vi "WSVCAP SHL FPGA LL Procedure SPI - Send Receive.vi"(0 "Procedure Step":T1, 1 "Wait Ticks Remaining":u32, 2 "CMD Length [1-40]":u8, 5 "SPI Wait Ticks":u32, 7 "Write Bit Index [0-39]":u8, 9 "SPI Cycle Mode":bool, 11 "error in (no error)":errorcluster, 12 "SPI Cycle CMD":u64, 13 "Socket Mask":u32) -> (3 "Wait Ticks Remaining Out":u32, 4 "Procedure Step Out":T1, 8 "Write Bit Index [0-39] Out":u8, 10 "Finished":bool, 15 "error out":errorcluster)   [LabVIEW 2012]
uses:
  Type Defs/WSVCAP SHL Procedure Step Enum.ctl
  Type Defs/WSVCAP SHL SPI Write Line Enum.ctl
  Type Defs/WSVCAP SHL FIFO Operation Enum.ctl
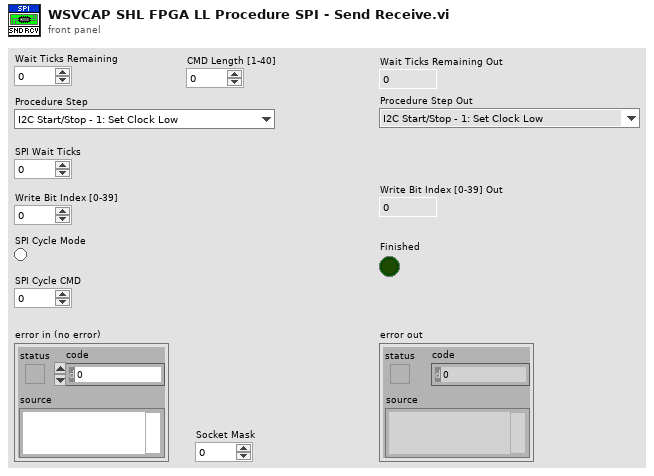
[diagram p1: front panel]
types:
  T1 = typedef "WSVCAP SHL Procedure Step Enum.ctl" = enum16{"I2C Start/Stop - 1: Set Clock Low", "I2C Start/Stop - 2: Wait", "I2C Start/Stop - 3: Set Data I", "I2C Start/Stop - 4: Wait", "I2C Start/Stop - 5: Set Clock High", "I2C Start/Stop - 6: Wait", "I2C Start/Stop - 7: Set Data II", "I2C Start/Stop - 8: Wait", "I2C Start/Stop - 9: Set Clock Low", "I2C Start/Stop - 10: Wait", "I2C Read ACK - 1: Set Clock High", "I2C Read ACK - 2: Wait", "I2C Read ACK - 3: Read ACK Bit", "I2C Read ACK - 4: Wait", "I2C Read ACK - 5: Set Clock Low", "I2C Read ACK - 6: Wait", "I2C Write ACK - 1: Write ACK Bit", "I2C Write ACK - 2: Wait", "I2C Write ACK - 3: Set Clock High", "I2C Write ACK - 4: Wait", "I2C Write ACK - 5: Set Clock Low", "I2C Write ACK - 6: Wait", "I2C Write ACK - 7: Set Data Low", "I2C Send Add - 1: Reset Bits Remaining", "I2C Send Add - 2: Set Data Bit", "I2C Send Add - 3: Wait", "I2C Send Add - 4: Set Clock High", "I2C Send Add - 5: Wait", "I2C Send Add - 6: Set Clock Low", "I2C Send Add - 7: Wait", "I2C Send Add - 8: Check Bits Remaining", "I2C Send Data - 1: Reset Bits Remaining", "I2C Send Data - 2: Load Write Bit from FIFO", "I2C Send Data - 3: Set Data Bit", "I2C Send Data - 4: Wait", "I2C Send Data - 5: Set Clock High", "I2C Send Data - 6: Wait", "I2C Send Data - 7: Set Clock Low", "I2C Send Data - 8: Wait", "I2C Send Data - 9: Check Bits Remaining", "I2C Receive Data - 1: Reset Bits Remaining", "I2C Receive Data - 2: Wait", "I2C Receive Data - 3: Set Clock High", "I2C Receive Data - 4: Wait", "I2C Receive Data - 5: Read Data Bit", "I2C Receive Data - 6: Wait", "I2C Receive Data - 7: Set Clock Low", "I2C Receive Data - 8: Wait", "I2C Receive Data - 9: Check Bits Remaining", "SPI Clear Lines - 1:Clear", "SPI Send/Receive - 1: Load SDA - Clock Low", "SPI Send/Receive - 2: Wait", "SPI Send/Receive - 3: Load DATO - Clock High", "SPI Send/Receive - 4: Wait", "SPI Wait CMD Delay - 1:Wait", "RFFE Send SSC - 1:Set Low", "RFFE Send SSC - 2:Wait", "RFFE Send SSC - 3:Set SDA High", "RFFE Send SSC - 4:Wait", "RFFE Send SSC - 5:Set SDA Low", "RFFE Send SSC - 6:Wait", "RFFE Send Data - 1:Set SCL High", "RFFE Send Data - 2:Wait", "RFFE Send Data - 3:Set SCL Low", "RFFE Send Data - 4:Wait", "RFFE Send Data - 5:Set SCL High (P)", "RFFE Send Data - 6:Wait", "RFFE Send Data - 7:Set SCL Low (P)", "RFFE Send Data - 8:Wait", "RFFE Send Data - 9:Set SCL High (BP)", "RFFE Send Data - 10:Wait", "RFFE Send Data - 11:Set SCL Low (BP)", "RFFE Send Data - 12:Wait", "RFFE Receive Data - 1:Set SCL High", "RFFE Receive Data - 2:Wait", "RFFE Receive Data - 3:Set SCL Low", "RFFE Receive Data - 4:Wait", "RFFE Receive Data - 5:Set SCL High (BP)", "RFFE Receive Data - 6:Wait", "RFFE Receive Data - 7:Set SCL Low (BP)", "RFFE Receive Data - 8:Wait", "RFFE Wait CMD Delay - 1:Wait", "RFFE Clear Lines - 1:Clear"}
  T2 = typedef "WSVCAP SHL SPI Write Line Enum.ctl" = enum16{"SDAA", "SDEN", "SCLK"}
  T3 = typedef "WSVCAP SHL FIFO Operation Enum.ctl" = enum16{"Create FIFO/Memory", "Get Write FIFO Status", "Get Read FIFO Status", "Put Element in Write", "Put Element in Read", "Get Element from Write", "Get Element from Read"}
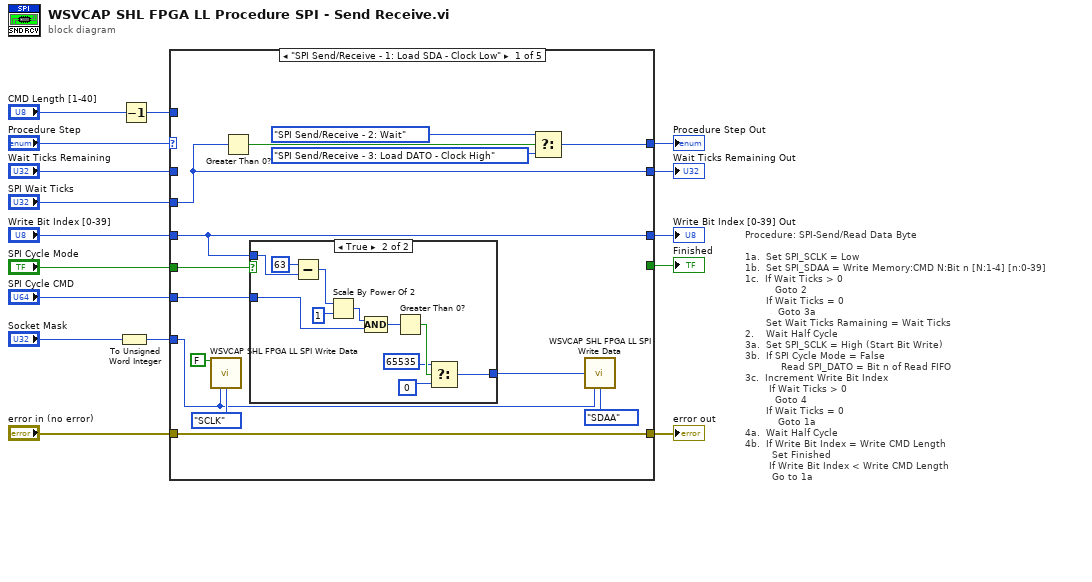
[diagram p0: block diagram]
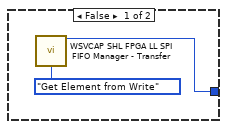
[diagram p2: hidden frame]
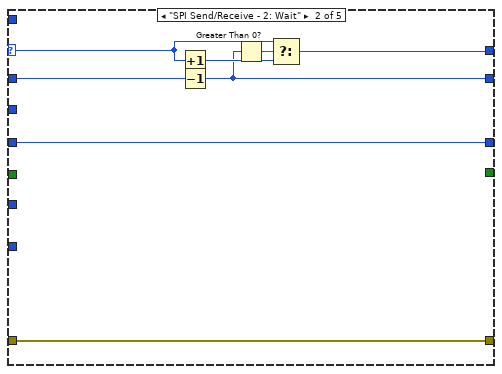
[diagram p3: hidden frame]
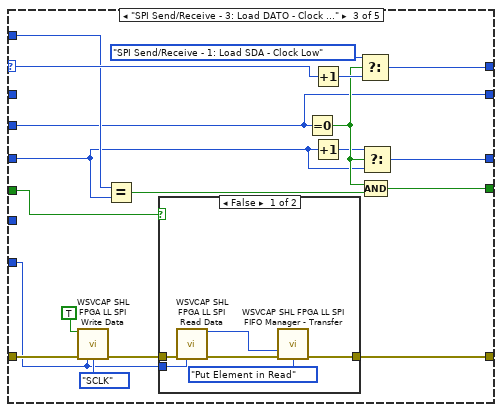
[diagram p4: hidden frame]
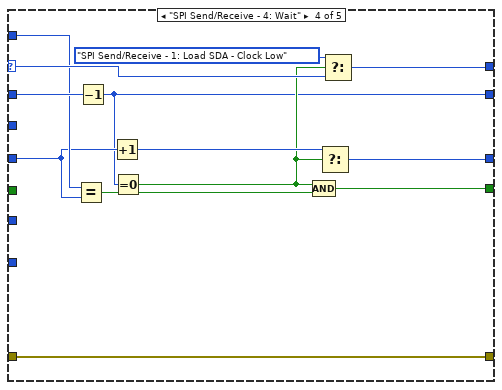
[diagram p6: hidden frame]
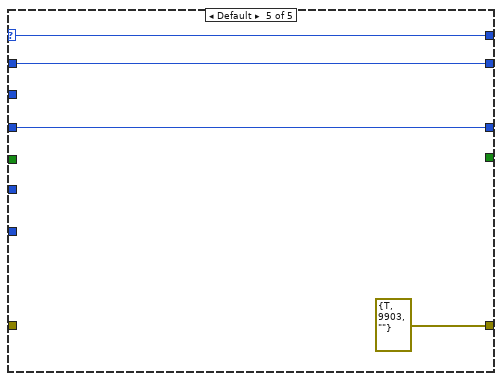
[diagram p7: hidden frame]
diagram:
  # "Procedure: SPI-Send/Read Data Byte\n\n1a.  Set SPI_SCLK = Low\n1b.  Set SPI_SDAA = Write Memory:CMD N:Bit n [N:1-4] [n:0-39]\n1c.  If Wait Ticks > 0\n          Goto 2\n       If Wait Ticks = 0 \n           Goto 3a\n       Set Wait Ticks Ramaining = Wait Ticks\n2.    Wait Half Cycle\n3a.  Set SPI_SCLK = High (Start Bit Write)\n3b.  If SPI Cycle Mode = False\n            Read SPI_DATO = Bit n of Read FIFO            \n3c.  Increment Write Bit Index\n        If Wait Ticks > 0\n          Goto 4\n       If Wait Ticks = 0 \n           Goto 1a \n4a.  Wait Half Cycle\n4b.  If Write Bit Index = Write CMD Length\n         Set Finished\n        If Write Bit Index < Write CMD Length\n         Go to 1a"
  n1 = To Unsigned Word Integer(number="Socket Mask") -> (unsigned 16bit integer=w11:u16)
  n2 = Decrement(x="CMD Length [1-40]") -> (x-1=w10:u8)
  n3 = case shown="\"SPI Send/Receive - 1: Load SDA - Clock Low\"" "Procedure Step" {
    selector: "Procedure Step" -> [_ w49 w70 w89 w93]
    tunnel: [w24 w51 w64 w90 errorcluster {"status"=TRUE, "code"=9903, "source"=""} ("error IO")] -> w15
    tunnel: "error in (no error)" -> [w24 w51 w66 w90 _]
    tunnel: "Wait Ticks Remaining" -> [_ w47 _ w88 w92]
    tunnel: "SPI Wait Ticks" -> [w18 _ w53 _ _]
    tunnel: [_ _ w62 w82 _] -> w14
    tunnel: "Write Bit Index [0-39]" -> [w17 w44 w56 w86 w91]
    tunnel: w11 -> [w26 _ w63 _ _]
    tunnel: "SPI Cycle Mode" -> [w23 _ w61 _ _]
    tunnel: "SPI Cycle CMD" -> [w22 _ _ _ _]
    tunnel: w10 -> [_ _ w60 w87 _]
    tunnel: [w19 w46 w54 w80 w93] -> w3
    tunnel: [w18 w45 w53 w79 w92] -> w2
    tunnel: [w17 w44 w52 w78 w91] -> w1
    frame "SPI Send/Receive - 1: Load SDA - Clock Low" {
      n4 = call "WSVCAP SHL FPGA LL SPI Write Data.vi"("Bit In"=FALSE, "Socket Mask"=w26, "Line"=WSVCAP_SHL_SPI_Write_Line_Enum."SCLK") -> ()  [unwired: 12 in, 1 out]
      n5 = Greater Than 0?(x=w18) -> (x > 0?=w27:bool)
      n6 = case shown="True" w23 {
        tunnel: [w31 w37] -> w25
        tunnel: w22 -> [_ w36]
        tunnel: w17 -> [_ w34]
        frame False {
          n7 = call "WSVCAP SHL FPGA LL SPI FIFO Manager - Transfer.vi"("Operation"=WSVCAP_SHL_FIFO_Operation_Enum."Get Element from Write") -> ("Data Out"=w31:u16)  [unwired: 12 in, 2 out]
        }
        frame True {
          n8 = Subtract(x=u8 63 ("y"), y=w34) -> (x-y=w33:u8)
          n9 = Scale By Power Of 2(n=w33, x=u64 1 ("Data Out")) -> (x*2^n=w42:u64)
          n10 = Compound Arithmetic op=AND(w42, w36) -> (w41:u64)
          n11 = Greater Than 0?(x=w41) -> (x > 0?=w40:bool)
          n12 = Select(t=u16 65535 ("Data Out"), s=w40, f=u16 0 ("Data Out")) -> (s? t:f=w37:u16)
        }
      }
      n13 = Select(t=WSVCAP_SHL_Procedure_Step_Enum."SPI Send/Receive - 2: Wait" ("Procedure Step"), s=w27, f=WSVCAP_SHL_Procedure_Step_Enum."SPI Send/Receive - 3: Load DATO - Clock High" ("Procedure Step")) -> (s? t:f=w19:T1)
      n14 = call "WSVCAP SHL FPGA LL SPI Write Data.vi"("Data Word In"=w25, "Socket Mask"=w26, "Line"=WSVCAP_SHL_SPI_Write_Line_Enum."SDAA") -> ()  [unwired: 12 in, 1 out]
    }
    frame "SPI Send/Receive - 2: Wait" {
      n15 = Increment(x=w49) -> (x+1=w48:T1)
      n16 = Decrement(x=w47) -> (x-1=w45:u32)
      n17 = Greater Than 0?(x=w45) -> (x > 0?=w50:bool)
      n18 = Select(t=w49, s=w50, f=w48) -> (s? t:f=w46:T1)
    }
    frame "SPI Send/Receive - 3: Load DATO - Clock High" {
      n19 = call "WSVCAP SHL FPGA LL SPI Write Data.vi"("Bit In"=TRUE, "error in (no error)"=w66, "Socket Mask"=w63, "Line"=WSVCAP_SHL_SPI_Write_Line_Enum."SCLK") -> ("error out"=w65:errorcluster)  [unwired: 11 in]
      n20 = Equal?(x=w60, y=w56) -> (x = y?=w59:bool)
      n21 = case shown="False" w61 {
        tunnel: w65 -> [w76 w77]
        tunnel: [w73 w77] -> w64
        tunnel: w63 -> [w72 _]
        frame False {
          n22 = call "WSVCAP SHL FPGA LL SPI Read Data.vi"("error in (no error)"=w76, "Socket Mask"=w72) -> ("Word Out (1-Bit for Each Channel)"=w71:u16, "error out"=w74:errorcluster)  [unwired: 12 in]
          n23 = call "WSVCAP SHL FPGA LL SPI FIFO Manager - Transfer.vi"("Word In"=w71, "error in (no error)"=w74, "Operation"=WSVCAP_SHL_FIFO_Operation_Enum."Put Element in Read") -> ("error out"=w73:errorcluster)  [unwired: 10 in, 2 out]
        }
        frame True {
        }
      }
      n24 = Equal To 0?(x=w53) -> (x = 0?=w58:bool)
      n25 = Increment(x=w70) -> (x+1=w69:T1)
      n26 = Increment(x=w56) -> (x+1=w57:u8)
      n27 = Select(t=WSVCAP_SHL_Procedure_Step_Enum."SPI Send/Receive - 1: Load SDA - Clock Low" ("Procedure Step"), s=w58, f=w69) -> (s? t:f=w54:T1)
      n28 = Select(t=w57, s=w58, f=w56) -> (s? t:f=w52:u8)
      n29 = Compound Arithmetic op=AND(w58, w59) -> (w62:bool)
    }
    frame "SPI Send/Receive - 4: Wait" {
      n30 = Equal?(x=w87, y=w86) -> (x = y?=w83:bool)
      n31 = Decrement(x=w88) -> (x-1=w79:u32)
      n32 = Increment(x=w86) -> (x+1=w85:u8)
      n33 = Equal To 0?(x=w79) -> (x = 0?=w84:bool)
      n34 = Compound Arithmetic op=AND(w84, w83) -> (w82:bool)
      n35 = Select(t=w85, s=w84, f=w86) -> (s? t:f=w78:u8)
      n36 = Select(t=WSVCAP_SHL_Procedure_Step_Enum."SPI Send/Receive - 1: Load SDA - Clock Low" ("Procedure Step"), s=w84, f=w89) -> (s? t:f=w80:T1)
    }
    frame Default {
    }
  }
  "error out" <- w15
  "Finished" <- w14
  "Procedure Step Out" <- w3
  "Wait Ticks Remaining Out" <- w2
  "Write Bit Index [0-39] Out" <- w1
